vi "Kaelus SWI Get Stimulus.vi"(7 "Summitek SWI":T4, 8 "error in (no error)":errorcluster, 11 "DAQmx Dev Name (SWModule)":string) -> (0 "error out":errorcluster, 3 "DAQmx Dev Name (SWModule)":string, 5 "SWI Position":T1)   [LabVIEW 2011]
uses:
  TypeDefs/Summitek SWI Position.ctl
  PIM/PIMHW/LIB/MODULES/SW Module/SW Tx Positions.ctl
  PIM/PIMHW/LIB/MODULES/SW Module/SW Rx Positions.ctl
  TypeDefs/Summitek SWI Instrument Info.ctl
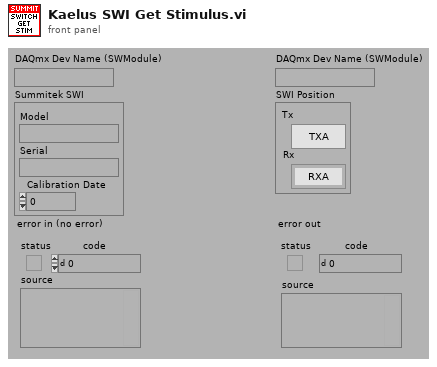
[diagram p1: front panel]
types:
  T1 = typedef "Summitek SWI Position.ctl" = cluster{"Tx":T2, "Rx":T3}
  T2 = typedef "SW Tx Positions.ctl" = enum16{"TXA", "TXB", "TXC"}
  T3 = typedef "SW Rx Positions.ctl" = enum16{"RXA", "RXB", "RXC", "RXD", "RXE", "RXF"}
  T4 = typedef "Summitek SWI Instrument Info.ctl" = cluster{"Model":string, "Serial":string, "Calibration Date":dbl}
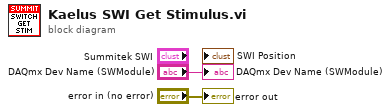
[diagram p0: block diagram]
diagram:
  "error out" <- "error in (no error)"
  "DAQmx Dev Name (SWModule)" <- "DAQmx Dev Name (SWModule)"
